vi "uTTA_Receive.vi"(7 "Timeout(ms)":i32, 8 "error in (no error)":errorcluster, 9 "Response Qualifier(\"\")":string, 10 "RX Termination(\\n)":string, 11 "VISA Refnum in":refnum<visa-resource-name>) -> (0 "error out":errorcluster, 1 "Response":string, 2 "Found response":bool, 3 "VISA Refnum out":refnum<visa-resource-name>)   [LabVIEW 2021]
uses:
  uTTA_GV_Serial_Monitor.vi
panel:
  out "Raw Received":string
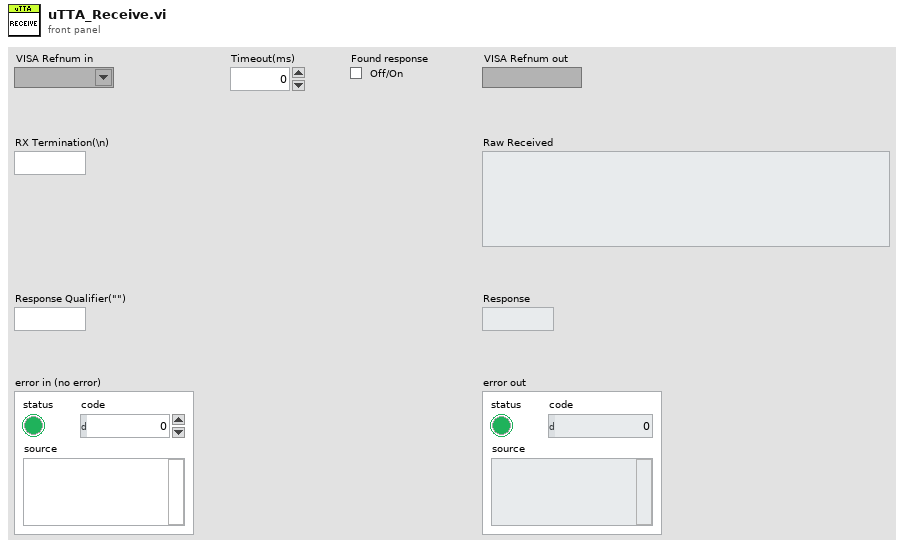
[diagram p1: front panel]
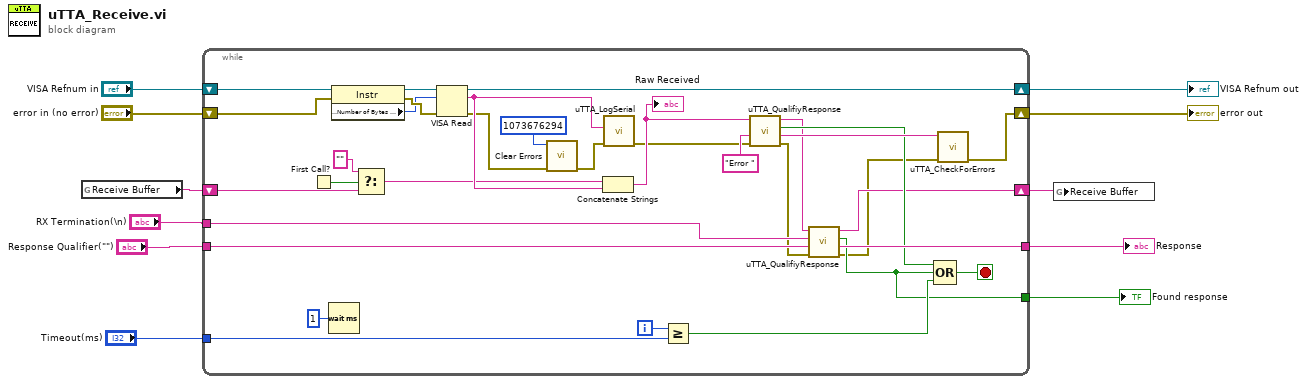
[diagram p0: block diagram]
diagram:
  n1 = global read "uTTA_GV_Serial_Monitor.vi" "Receive Buffer"() -> (w2:string)
  n2 = while {
    shift-right: [w13] -> w1
    shift-left: w2 -> [w31]
    shift-right: [w35] -> w11
    shift-left: "error in (no error)" -> [w43]
    shift-right: [w38] -> w8
    shift-left: "VISA Refnum in" -> [w44]
    tunnel: "Timeout(ms)" -> [w36]
    tunnel: "RX Termination(\\n)" -> [w27]
    tunnel: "Response Qualifier(\"\")" -> [w33]
    tunnel: [w28] -> w7
    tunnel: [w18] -> w9
    i -> [w37]
    stop <- w22 stop-if-true
    n3 = First Call?() -> (First Call?: T/F=w32:bool)
    n4 = Wait (ms)(milliseconds to wait=u32 1) -> ()  [unwired: 1 out]
    n5 = property class="Instr"(reference=w44, error in=w43) -> (reference out=w42:refnum<visa-resource-name>, error out=w41:errorcluster, "Serial Settings:Number of Bytes at Serial Port"=w40:u32)
    n6 = Select(t="", s=w32, f=w31) -> (s? t:f=w30:string)
    n7 = VISA Read(VISA resource name=w42, byte count=w40, error in (no error)=w41) -> (VISA resource name out=w38:refnum<visa-resource-name>, read buffer=w34:string, error out=w20:errorcluster)  [unwired: 1 out]
    n8 = call <vilib>:"Clear Errors.vi"("error in (no error)"=w20, "specific error code to clear (0: all)"=1073676294) -> ("error out"=w19:errorcluster)  [unwired: 4 in, 1 out]
    n9 = Concatenate Strings(w30, w34) -> (w17:string)
    "Raw Received" <- w17
    n10 = call "uTTA_LogSerial.vi"("error in"=w19, "Data_Sent"=w34) -> ("error out"=w16:errorcluster)  [unwired: 5 in]
    n11 = Greater Or Equal?(x=w37, y=w36) -> (x >= y?=w23:bool)
    n12 = call "uTTA_QualifiyResponse.vi"("error in"=w16, "Response Qualifier(\"\")"="Error " ("Response Qualifier(\"\")"), "Databuffer IN"=w17) -> ("error out"=w14:errorcluster, "Response"=w25:string, "Found response"=w24:bool, "DataBuffer out"=w15:string)  [unwired: 1 in]
    n13 = call "uTTA_QualifiyResponse.vi"("error in"=w14, "Response Qualifier(\"\")"=w33, "RX Termination(\\n)"=w27, "Databuffer IN"=w15) -> ("error out"=w12:errorcluster, "Response"=w28:string, "Found response"=w18:bool, "DataBuffer out"=w13:string)
    n14 = Compound Arithmetic op=OR(w24, w18, w23) -> (w22:bool)
    n15 = call "uTTA_CheckForErrors.vi"("error in"=w12, "Received"=w25) -> ("error out"=w35:errorcluster)  [unwired: 9 in]
  }
  "error out" <- w11
  "Found response" <- w9
  "VISA Refnum out" <- w8
  "Response" <- w7
  n16 = global write "uTTA_GV_Serial_Monitor.vi" "Receive Buffer"(w1) -> ()
